vi "Place HDI.vi"(8 "error in":errorcluster, 9 "Slot Number":i32, 10 "Chuck Number":i32, 11 "PickupTool in":refnum<class "PickerTool Class.lvclass">) -> (0 "error out":errorcluster, 3 "PickupTool out":refnum<class "PickerTool Class.lvclass">)   [LabVIEW 2011, in "PickerTool Class.lvclass"]
uses:
  PickerTool Class.lvclass
  Config Manager Class/Type Definitions/Offset.ctl
  WorkTable Class/WorkTable Class.lvclass
  Vec3d Class/Vec3d Class.lvclass
  Config Manager Class/Config Manager Class.lvclass
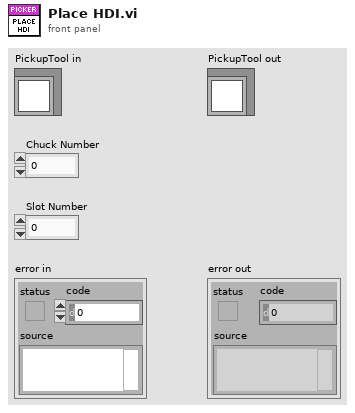
[diagram p1: front panel]
types:
  T1 = typedef "Offset.ctl" = enum16{"needle_offset", "tool_holder_offset"}
  T2 = typedef "Worktable_Module Slot.ctl" = cluster{"Slot State":enum16{"Empty", "Unglued", "Stamped", "PartOnTop", "Weighted", "Unpotted", "Potted"}, "BBM Type":enum16{"None", "BBM", "GlassSlide"}, "HDI Type":enum16{"None", "HDI", "Polyimide"}, "Vacuum Channel":u8, "Location/Orientation BBM":T3, "Location/Orientation HDI":T3, "S/N":string}
  T3 = typedef "Position_Orientation.ctl" = cluster{"Center":refnum<class "Vec3d Class.lvclass">, "Orientation":refnum<class "Orient3d Class.lvclass">}
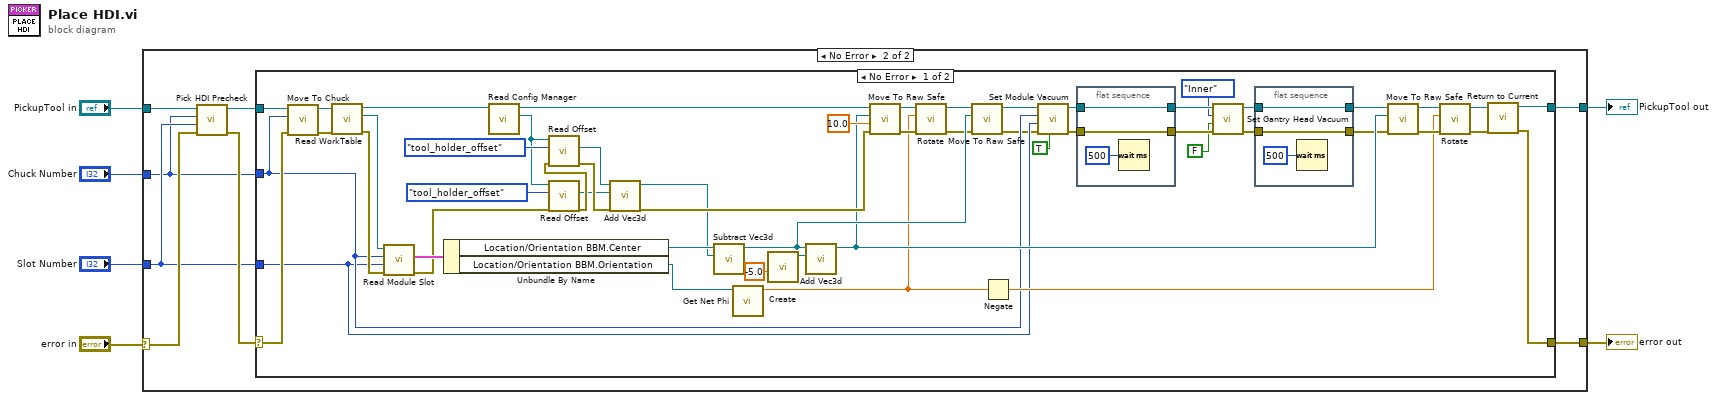
[diagram p0: block diagram]
diagram:
  n1 = case shown="No Error" "error in" {
    selector: "error in" -> [w7 w15]
    tunnel: [w7 w14] -> w5
    tunnel: [w8 w13] -> w6
    tunnel: "PickupTool in" -> [w8 w16]
    tunnel: "Slot Number" -> [_ w10]
    tunnel: "Chuck Number" -> [_ w9]
    frame Error {
    }
    frame No Error {
      n2 = call "Pick HDI Precheck.vi"("error in"=w15, "Slot Number in"=w10, "Chuck Number in"=w9, "PickupTool Class in"=w16) -> ("error out"=w11:errorcluster, "PickupTool Class out"=w12:refnum<class "PickerTool Class.lvclass">)  [unwired: 6 in]
      n3 = case shown="No Error" w11 {
        selector: w11 -> [w68 w77]
        tunnel: [w43 w77] -> w14
        tunnel: w12 -> [w69 w76]
        tunnel: [w44 w76] -> w13
        tunnel: w10 -> [w26 _]
        tunnel: w9 -> [w27 _]
        frame No Error {
          n4 = call-dynamic "Move To Chuck.vi"("error in"=w68, "Chuck"=w27, "Gantry in"=w69) -> ("error out"=w57:errorcluster, "Gantry out"=w61:refnum<class "PickerTool Class.lvclass">)  [unwired: 7 in]
          n5 = call-dynamic "Read WorkTable.vi"("error in"=w57, "Gantry Class in"=w61) -> ("error out"=w66:errorcluster, "WorkTable Class.lvclass"=w67:refnum<class "WorkTable Class.lvclass">, "Gantry Class out"=w60:refnum<class "PickerTool Class.lvclass">)  [unwired: 7 in]
          n6 = call-dynamic "Read Module Slot.vi"("error in"=w66, "slot"=w26, "chuck"=w27, "WorkTable in"=w67) -> ("error out"=w55:errorcluster, "Module Slot"=w65:T2)  [unwired: 5 in, 1 out]
          n7 = Unbundle By Name(w65) -> ("Location/Orientation BBM.Center"=w50:refnum<class "Vec3d Class.lvclass">, "Location/Orientation BBM.Orientation"=w42:refnum<class "Orient3d Class.lvclass">)
          n8 = call-dynamic "Read Config Manager.vi"("Gantry in"=w60) -> ("Config Manager"=w56:refnum<class "Config Manager Class.lvclass">, "Gantry out"=w59:refnum<class "PickerTool Class.lvclass">)  [unwired: 8 in, 1 out]
          n9 = call "Read Offset.vi"("error in"=w55, "Offset"=Offset."tool_holder_offset", "Config Manager in"=w56) -> ("error out"=w54:errorcluster, "Vec3d out"=w51:refnum<class "Vec3d Class.lvclass">)  [unwired: 6 in, 1 out]
          n10 = call "Read Offset.vi"("error in"=w54, "Offset"=Offset."tool_holder_offset", "Config Manager in"=w56) -> ("error out"=w53:errorcluster, "Vec3d out"=w64:refnum<class "Vec3d Class.lvclass">)  [unwired: 6 in, 1 out]
          n11 = call-dynamic "Add Vec3d.vi"("error in (no error)"=w53, 10:"Vec3d Class in"=w51, 11:"Vec3d Class in"=w64) -> ("error out"=w62:errorcluster, "Vec3d Class out"=w49:refnum<class "Vec3d Class.lvclass">)  [unwired: 7 in]
          n12 = call "Subtract Vec3d.vi"("Vec3d in 2"=w49, "Vec3d in 1"=w50) -> ("Vec3d Class out"=w46:refnum<class "Vec3d Class.lvclass">)  [unwired: 8 in, 1 out]
          n13 = call "Get Net Phi.vi"("Orient3d"=w42) -> ("phi(deg)"=w17:dbl)  [unwired: 8 in, 2 out]
          n14 = call "Create.vi"("Z"=-5.0) -> ("Vec3d Class out"=w47:refnum<class "Vec3d Class.lvclass">)  [unwired: 9 in, 1 out]
          n15 = call-dynamic "Add Vec3d.vi"(10:"Vec3d Class in"=w47, 11:"Vec3d Class in"=w46) -> ("Vec3d Class out"=w45:refnum<class "Vec3d Class.lvclass">)  [unwired: 8 in, 1 out]
          n16 = call-dynamic "Move To Raw Safe.vi"("error in"=w62, "Speed(mm/s)"=10.0 ("Speed"), "Destination"=w45, "Gantry in"=w59) -> ("error out"=w39:errorcluster, "Gantry out"=w41:refnum<class "PickerTool Class.lvclass">)  [unwired: 6 in]
          n17 = call-dynamic "Rotate.vi"("error in"=w39, "distance(deg)"=w17, "Gantry in"=w41) -> ("error out"=w38:errorcluster, "Gantry out"=w40:refnum<class "PickerTool Class.lvclass">)  [unwired: 7 in]
          n18 = call-dynamic "Move To Raw Safe.vi"("error in"=w38, "Destination"=w46, "Gantry in"=w40) -> ("error out"=w25:errorcluster, "Gantry out"=w29:refnum<class "PickerTool Class.lvclass">)  [unwired: 7 in]
          n19 = Negate(x=w17) -> (-x=w33:dbl)
          n20 = call-dynamic "Set Module Vacuum.vi"("On/Off"=TRUE, "error in"=w25, "Slot Number"=w26, "Chuck Number"=w27, "Gantry in"=w29) -> ("error out"=w18:errorcluster, "Gantry out"=w30:refnum<class "PickerTool Class.lvclass">)  [unwired: 5 in]
          n21 = flat-sequence {
            tunnel: w30 -> [w72]
            tunnel: [w72] -> w24
            tunnel: w18 -> [w71]
            tunnel: [w71] -> w21
            frame #0 {
              n22 = Wait (ms)(milliseconds to wait=u32 500) -> ()  [unwired: 1 out]
            }
          }
          n23 = call-dynamic "Set Gantry Head Vacuum.vi"("error in (no error)"=w21, "On/Off"=FALSE, "Inner/Outer"=enum16{"Outer", "Inner"}."Inner", "Gantry Class in"=w24) -> ("error out"=w22:errorcluster, "Gantry Class out"=w23:refnum<class "PickerTool Class.lvclass">)  [unwired: 6 in]
          n24 = flat-sequence {
            tunnel: w23 -> [w75]
            tunnel: [w75] -> w32
            tunnel: w22 -> [w74]
            tunnel: [w74] -> w31
            frame #0 {
              n25 = Wait (ms)(milliseconds to wait=u32 500) -> ()  [unwired: 1 out]
            }
          }
          n26 = call-dynamic "Move To Raw Safe.vi"("error in"=w31, "Destination"=w45, "Gantry in"=w32) -> ("error out"=w35:errorcluster, "Gantry out"=w37:refnum<class "PickerTool Class.lvclass">)  [unwired: 7 in]
          n27 = call-dynamic "Rotate.vi"("error in"=w35, "distance(deg)"=w33, "Gantry in"=w37) -> ("error out"=w34:errorcluster, "Gantry out"=w36:refnum<class "PickerTool Class.lvclass">)  [unwired: 7 in]
          n28 = call-dynamic "Return to Current.vi"("error in"=w34, "Gantry in"=w36) -> ("error out"=w43:errorcluster, "Gantry out"=w44:refnum<class "PickerTool Class.lvclass">)  [unwired: 8 in]
        }
        frame Error {
        }
      }
    }
  }
  "error out" <- w5
  "PickupTool out" <- w6
